vi "Get settings chain.vi"(8 "error in (no error)":errorcluster, 11 "TomoConversionBase in":refnum<class "TomoConversion.lvclass">) -> (0 "error out":errorcluster, 1 "class name":string[](array[string]), 2 "settings":variant[](array[variant]), 3 "TomoConversionBase out":refnum<class "TomoConversion.lvclass">)   [LabVIEW 2012, in "TomoConversion.lvclass"]
doc: "Returns an array of variants containing the settings clusters of each class in the inheritance chain (lowest child class first), together with an array of all class names in the inheritance chain.\n\nFor classes without settings cluster, the settings chain contains empty variants."
uses:
  TomoConversion.lvclass
  <vilib>/Distrio/Murmex/Murmex/Murmex.lvclass
  TomoConversion.lvclass/TomoConversion.ctl
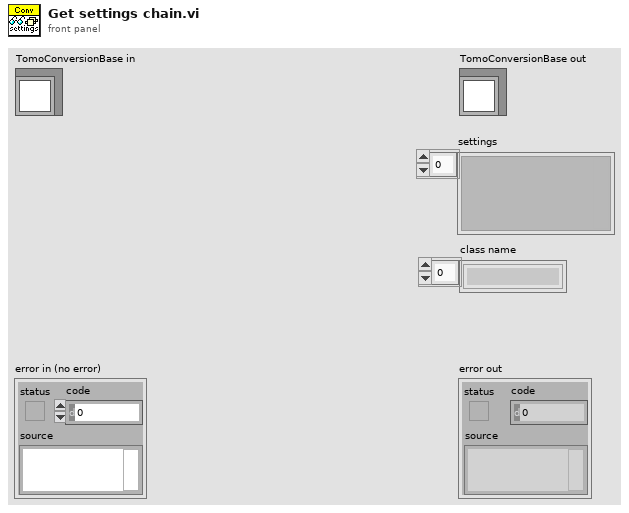
[diagram p1: front panel]
types:
  T1 = typedef "TomoConversion.lvclass/Settings_cluster.ctl" = cluster{"Slice per tiff file":u32, "Delete cxd file?":bool, "2x2 downsampling?":bool, "small volume z downsampling":i32, "small volume xy downsampling":T2}
  T2 = typedef "TomoConversion.lvclass/small volume downsampling.ctl" = i32
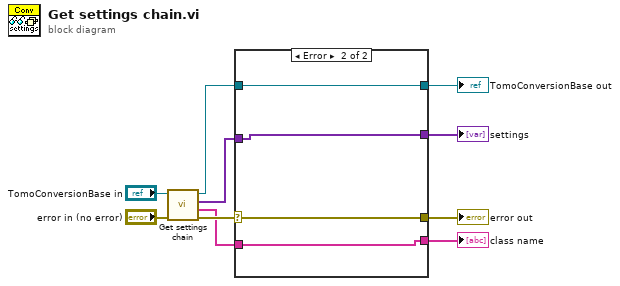
[diagram p0: block diagram]
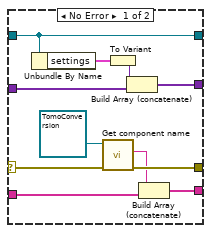
[diagram p2: hidden frame]
diagram:
  n1 = call-parent "Get settings chain.vi"("error in (no error)"="error in (no error)", "MurmexBase in"="TomoConversionBase in") -> ("error out"=w8:errorcluster, "class name"=w6:string[], "settings"=w4:variant[], "MurmexBase out"=w3:refnum<class "TomoConversion.lvclass">)  [unwired: 6 in]
  n2 = case shown="Error" w8 {
    selector: w8 -> [w21 w24]
    tunnel: [w20 w24] -> w7
    tunnel: w6 -> [w18 w25]
    tunnel: [w16 w25] -> w5
    tunnel: w4 -> [w15 w23]
    tunnel: w3 -> [w12 w22]
    tunnel: [w12 w22] -> w2
    tunnel: [w11 w23] -> w1
    frame No Error {
      n3 = Unbundle By Name(w12) -> ("settings"=w13:T1)
      n4 = call <vilib>:"Get component name.vi"("error in (no error)"=w21, "Murmex in"=refnum<class "TomoConversion.lvclass"> refnum ("TomoConversion.lvclass")) -> ("error out"=w20:errorcluster, "component name"=w17:string)  [unwired: 7 in, 1 out]
      n5 = To Variant(anything=w13) -> (Variant=w14:variant)
      n6 = Build Array (concatenate)(w14, w15) -> (w11:variant[])
      n7 = Build Array (concatenate)(w17, w18) -> (w16:string[])
    }
    frame Error {
    }
  }
  "error out" <- w7
  "TomoConversionBase out" <- w2
  "settings" <- w1
  "class name" <- w5
